vi "Drive freq to RPM.vi"(1 "Drive address":T1=1 items=["0", "1", "2", "3", "4", "5", "6", "7", "8", "9", "10", "11", "12", "13", "14", "15", "16", "17", "18", "19", "20", "21", "22", "23", "24", "25", "26", "27", "28", "29", "30", "31", "32", "33", "34", "35", "36", "37", "38", "39", "40", "41", "42", "43", "44", "45", "46", "47", "48", "49", "50", "51", "52", "53", "54", "55", "56", "57", "58", "59", "60", "61", "62", "63"], 2 "Drive output f (Hz)":dbl) -> (0 "Motor RPM (/min)":dbl)   [LabVIEW 2020]
doc: "Modbus RTU for Invertek drives. Paul Nathan 19-JUN-2022."
uses:
  ctls/Drive address.ctl
  Globals/Invertek Drive Params.vi
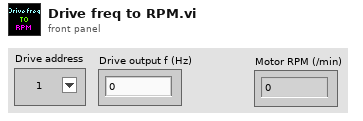
[diagram p1: front panel]
types:
  T1 = typedef "Drive address.ctl" = u8
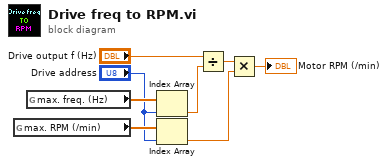
[diagram p0: block diagram]
diagram:
  n1 = global read "Invertek Drive Params.vi" "max. RPM (/min)"() -> (w5:dbl[])
  n2 = global read "Invertek Drive Params.vi" "max. freq. (Hz)"() -> (w4:dbl[])
  n3 = Index Array(array=w4, index="Drive address") -> (element=w2:dbl)
  n4 = Index Array(array=w5, index="Drive address") -> (element=w1:dbl)
  n5 = Divide(x="Drive output f (Hz)", y=w2) -> (x/y=w8:dbl)
  n6 = Multiply(x=w8, y=w1) -> (x*y=→"Motor RPM (/min)":dbl)
